vi "Send.vi"(6 "Severity Code (info)":T1=enum."info", 8 "Error In":errorcluster, 9 "Message Content":string, 10 "Message Tag":string, 11 "CS++MessageLogger in":refnum<class "CS++MessageLogger.lvclass">) -> (0 "Error Out":errorcluster, 3 "CS++MessageLogger out":refnum<class "CS++MessageLogger.lvclass">)   [LabVIEW 2016, in "CS++BaseClasses.lvlib" / "CS++MessageLogger.lvclass"]
doc: "Send mesage to message logger."
uses:
  CS++MessageLogger.lvclass
  Libraries/Base/Severity.ctl
  Libraries/Base/CS++Base.lvlib
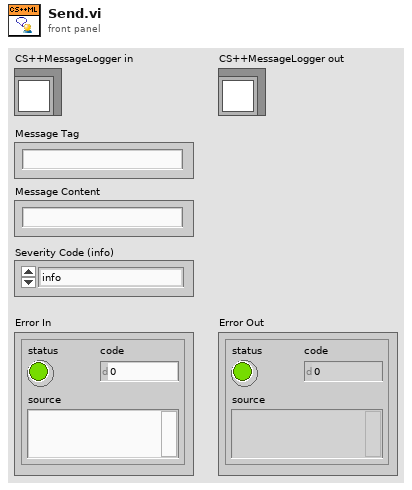
[diagram p1: front panel]
types:
  T1 = typedef "CS++Base.lvlib/Severity.ctl" = enum16{"emergency", "alert", "critical", "error", "warning", "notice", "info", "debug"}
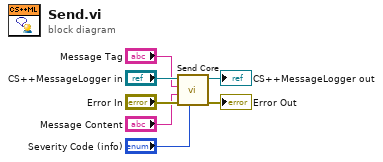
[diagram p0: block diagram]
diagram:
  n1 = call-dynamic "Send Core.vi"("Severity Code (info)"="Severity Code (info)", "Error In"="Error In", "Message Content"="Message Content", "Message Tag"="Message Tag", "CS++MessageLogger in"="CS++MessageLogger in") -> ("Error Out"=→"Error Out":errorcluster, "CS++MessageLogger out"=→"CS++MessageLogger out":refnum<class "CS++MessageLogger.lvclass">)  [unwired: 5 in]
